vi "enum2deg.vi"(9 "Rotation":T1) -> (1 "number":i32)   [LabVIEW 2020]
uses:
  Controls/Aug_Rotation.ctl
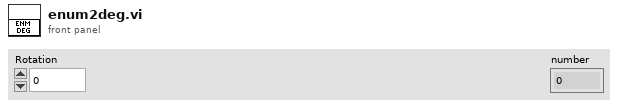
[diagram p1: front panel]
types:
  T1 = typedef "Aug_Rotation.ctl" = enum16{"0", "90", "180", "270"}
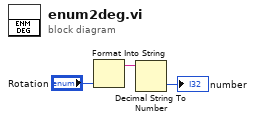
[diagram p0: block diagram]
diagram:
  n1 = Format Into String("Rotation") -> (resulting string=w2:string)  [unwired: 3 in, 1 out]
  n2 = Decimal String To Number(string=w2) -> (number=→"number":i32)  [unwired: 2 in, 1 out]
